vi "TLB Native Dynamic Events ver 0.02.vi"() -> ()   [LabVIEW 2018]
uses:
  Labview Training Phase 2/Enum Controls/States for Action Engine.ctl
panel:
  out "QUEUE OUTPUT":string
  in  "Stop Queue":bool
  in  "Start Queue":bool
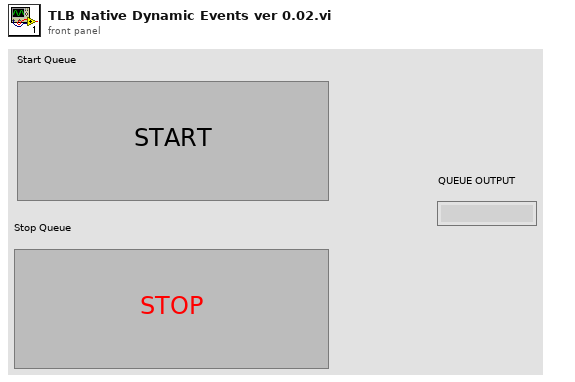
[diagram p1: front panel]
types:
  T1 = typedef "States for Action Engine.ctl" = enum16{"Initialize", "Write", "Read"}
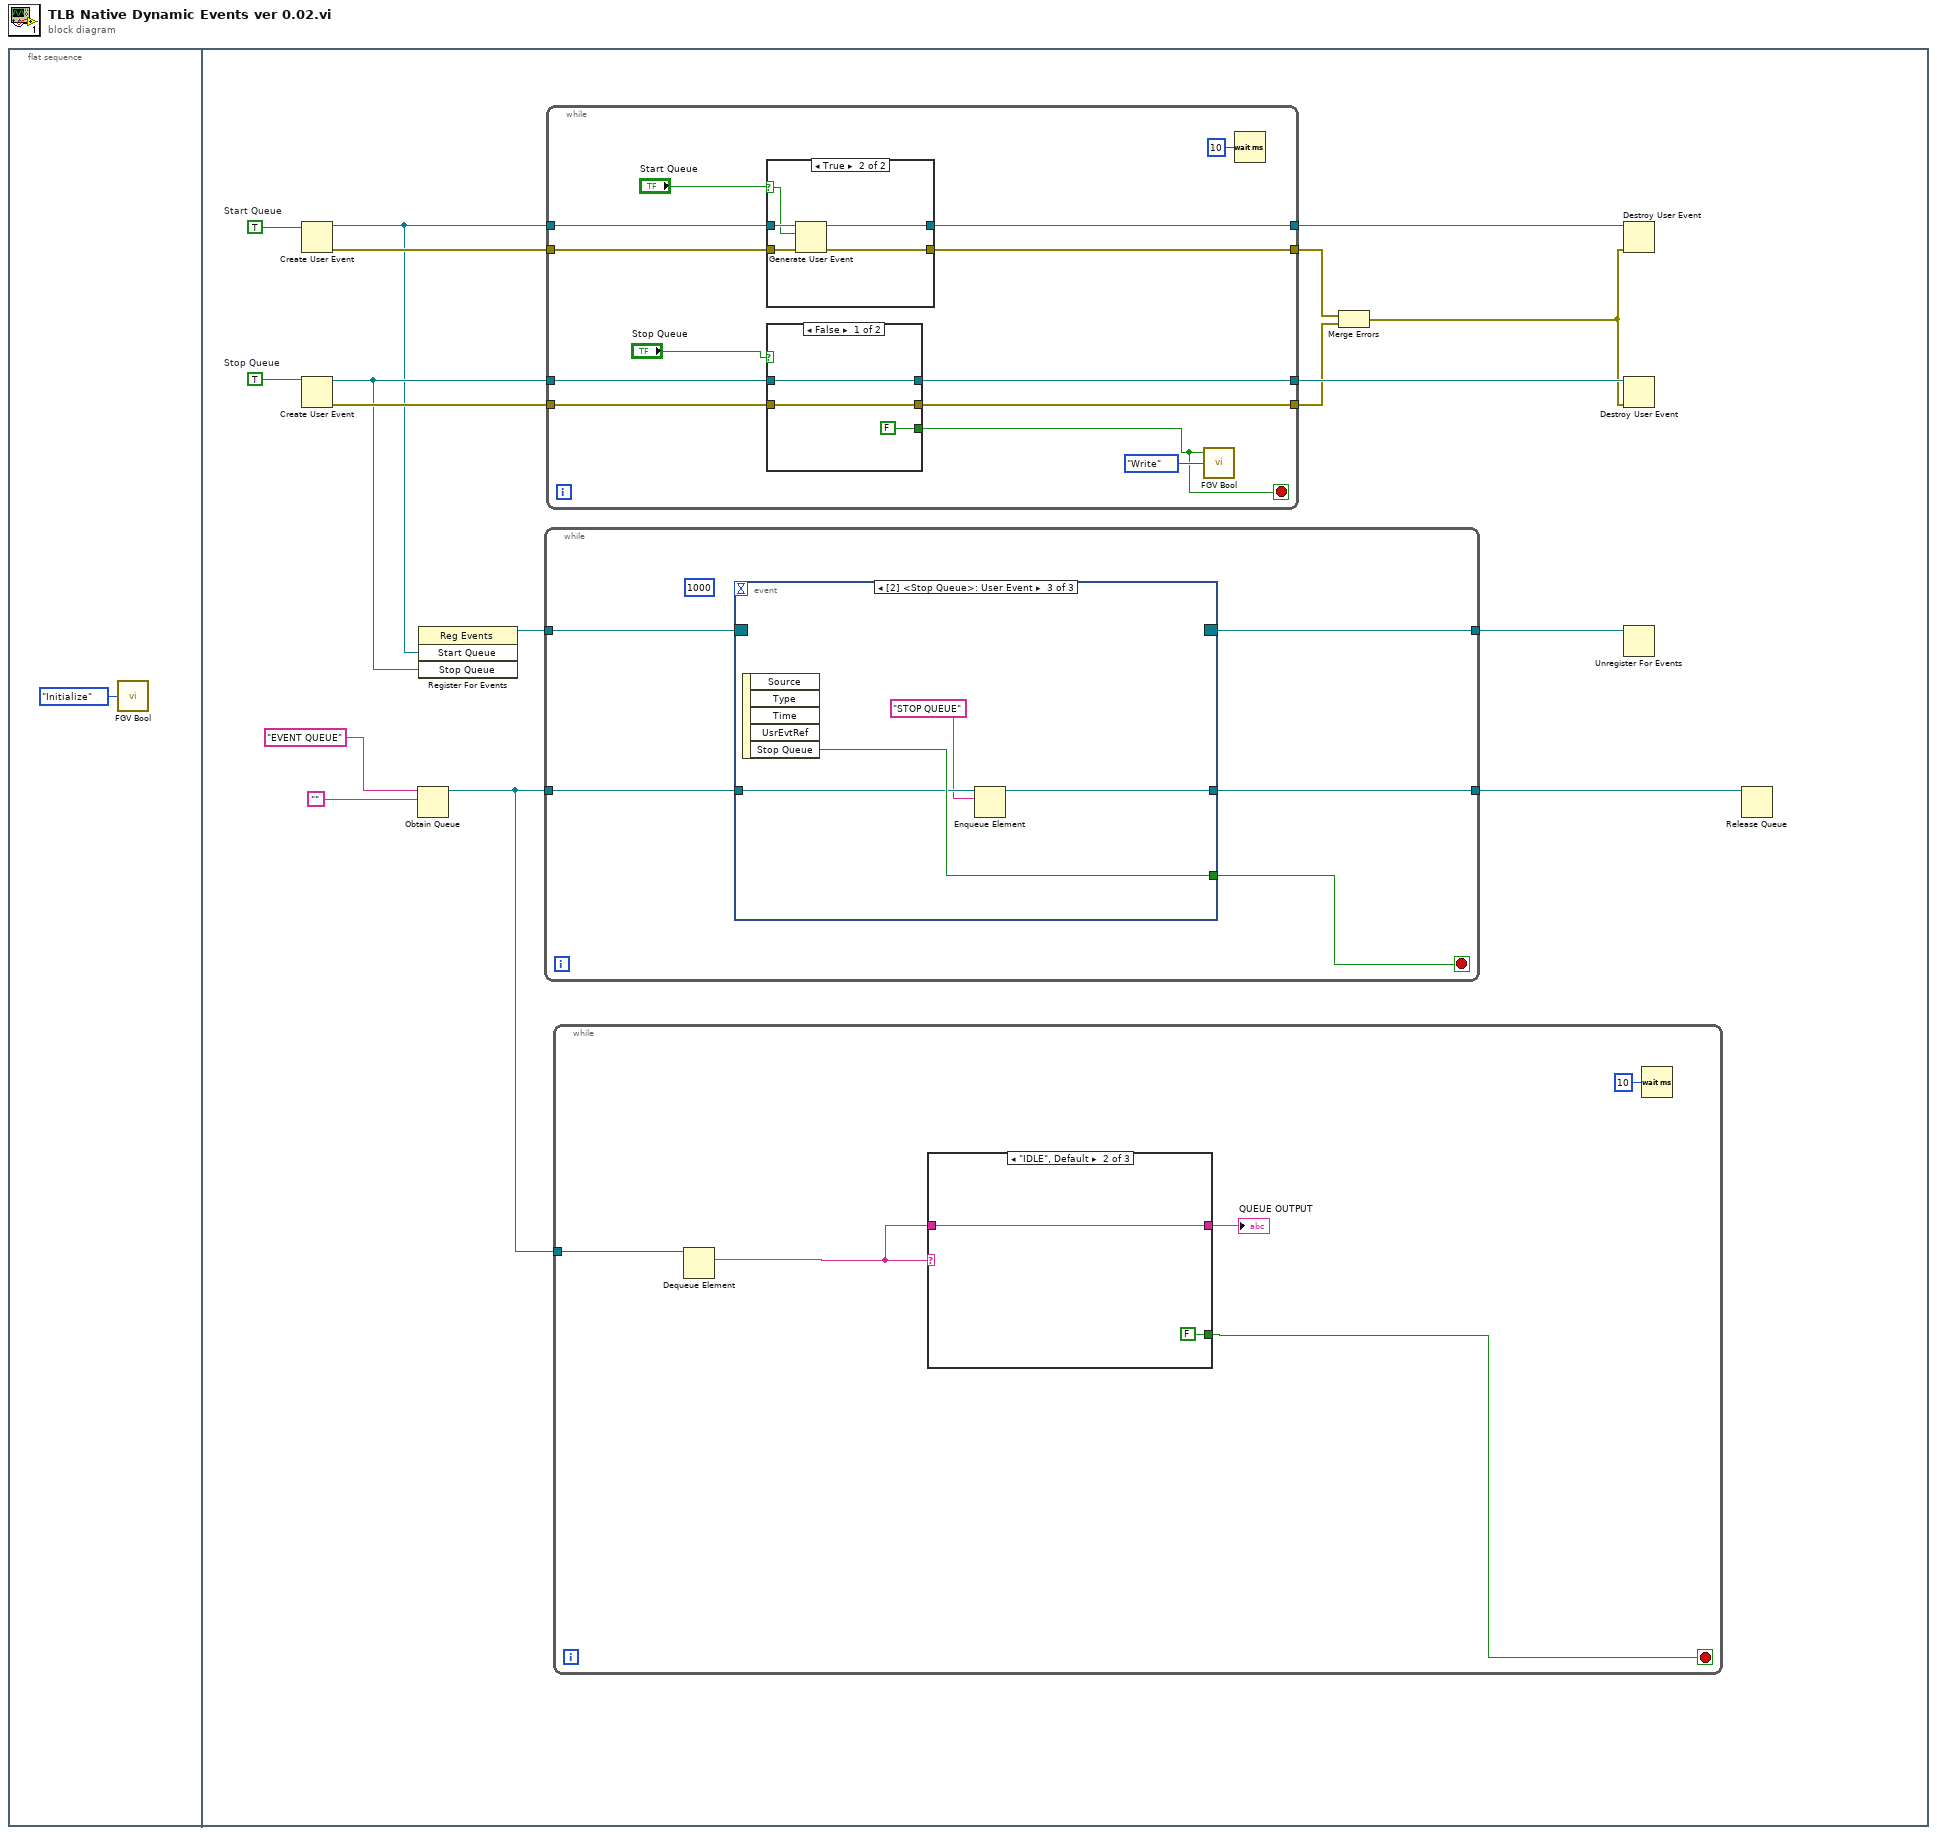
[diagram p0: block diagram]
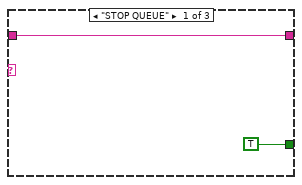
[diagram p2: hidden frame]
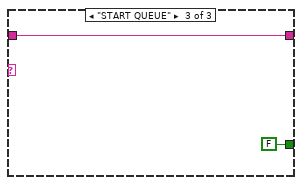
[diagram p3: hidden frame]
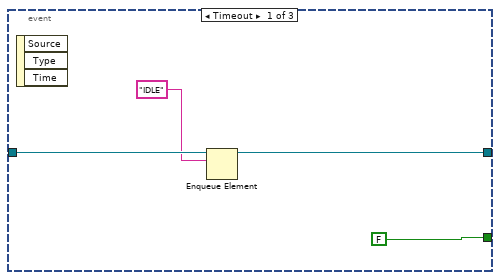
[diagram p4: hidden frame]
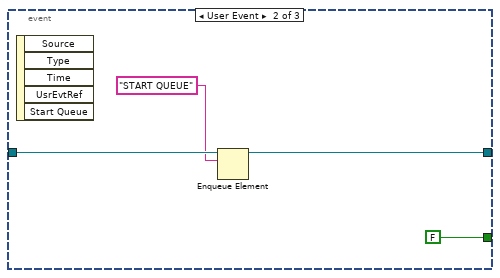
[diagram p5: hidden frame]
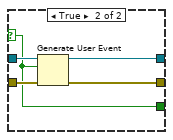
[diagram p6: hidden frame]
diagram:
  n1 = flat-sequence {
    frame #0 {
      n2 = call "FGV Bool.vi"("Init/Read/Write State"=States_for_Action_Engine."Initialize") -> ()  [unwired: 2 in, 2 out]
    }
    frame #1 {
      w18 = TRUE  # Stop Queue
      w17 = TRUE  # Start Queue
      n3 = Create User Event(user event datatype=w17) -> (user event=w8:refnum<user-event>, error out=w14:errorcluster)  [unwired: 1 in]
      n4 = Create User Event(user event datatype=w18) -> (user event=w9:refnum<user-event>, error out=w13:errorcluster)  [unwired: 1 in]
      n5 = Obtain Queue(name (unnamed)="EVENT QUEUE", element data type="") -> (queue out=w2:refnum<queue>)  [unwired: 3 in, 2 out]
      n6 = register-events(w8, w9) -> (reference out=w7:refnum<event-registration>)  [unwired: 2 in, 1 out]
      n7 = while {
        tunnel: w7 -> [w34]
        tunnel: [w33] -> w6
        tunnel: w2 -> [w31]
        tunnel: [w30] -> w5
        stop <- w32 stop-if-true
        (unwired) 1000
        n8 = event shown="[2] <Stop Queue>: User Event" {
          selector: w34 -> [_ _ _]
          dyn-events: [_ _ _] -> w33
          timeout: _ -> [_ _ _]
          tunnel: [FALSE FALSE w46] -> w32
          tunnel: w31 -> [w37 w41 w44]
          tunnel: [w36 w40 w45] -> w30
          event Timeout {
            n9 = event-data() -> ()  [unwired: 1 in, 3 out]
            n10 = Enqueue Element(queue=w37, element="IDLE") -> (queue out=w36:refnum<queue>)  [unwired: 2 in, 2 out]
          }
          event User Event {
            n11 = event-data() -> ()  [unwired: 1 in, 5 out]
            n12 = Enqueue Element(queue=w41, element="START QUEUE" ("name (unnamed)")) -> (queue out=w40:refnum<queue>)  [unwired: 2 in, 2 out]
          }
          event User Event {
            n13 = event-data() -> ("Stop Queue"=w46:bool)  [unwired: 1 in, 4 out]
            n14 = Enqueue Element(queue=w44, element="STOP QUEUE") -> (queue out=w45:refnum<queue>)  [unwired: 2 in, 2 out]
          }
        }
      }
      n15 = while {
        tunnel: w8 -> [w58]
        tunnel: w9 -> [w57]
        tunnel: [w56] -> w16
        tunnel: [w55] -> w15
        tunnel: w14 -> [w54]
        tunnel: [w53] -> w12
        tunnel: w13 -> [w52]
        tunnel: [w51] -> w11
        stop <- w47 stop-if-true
        n16 = case shown="True" "Start Queue" {
          selector: "Start Queue" -> [_ w70]
          tunnel: w58 -> [w69 w74]
          tunnel: [w69 w73] -> w55
          tunnel: w54 -> [w68 w72]
          tunnel: [w68 w71] -> w53
          frame False {
          }
          frame True {
            n17 = Generate User Event(user event=w74, event data cluster=w70, error in=w72) -> (user event out=w73:refnum<user-event>, error out=w71:errorcluster)  [unwired: 1 in]
          }
        }
        n18 = case shown="False" "Stop Queue" {
          selector: "Stop Queue" -> [_ w63]
          tunnel: w57 -> [w62 w67]
          tunnel: [w62 w66] -> w56
          tunnel: w52 -> [w61 w65]
          tunnel: [w61 w64] -> w51
          tunnel: [FALSE w63] -> w47
          frame False {
          }
          frame True {
            n19 = Generate User Event(user event=w67, event data cluster=w63, error in=w65) -> (user event out=w66:refnum<user-event>, error out=w64:errorcluster)  [unwired: 1 in]
          }
        }
        n20 = call "FGV Bool.vi"("Init/Read/Write State"=States_for_Action_Engine."Write", "Input Node"=w47) -> ()  [unwired: 1 in, 2 out]
        n21 = Wait (ms)(milliseconds to wait=u32 10) -> ()  [unwired: 1 out]
      }
      n22 = while {
        tunnel: w2 -> [w23]
        stop <- w19 stop-if-true
        n23 = Dequeue Element(queue=w23) -> (element=w22:string)  [unwired: 2 in, 3 out]
        n24 = case shown="\"IDLE\", Default" w22 {
          tunnel: w22 -> [w25 w27 w29]
          tunnel: [w25 w27 w29] -> w21
          tunnel: [TRUE FALSE FALSE] -> w19
          frame "STOP QUEUE" {
          }
          frame "IDLE", Default {
          }
          frame "START QUEUE" {
          }
        }
        "QUEUE OUTPUT" <- w21
        n25 = Wait (ms)(milliseconds to wait=u32 10) -> ()  [unwired: 1 out]
      }
      n26 = Merge Errors(w12, w11) -> (w10:errorcluster)
      n27 = Destroy User Event(user event=w15, error in=w10) -> ()  [unwired: 1 out]
      n28 = Destroy User Event(user event=w16, error in=w10) -> ()  [unwired: 1 out]
      n29 = Unregister For Events(event registration refnum=w6) -> ()  [unwired: 1 in, 1 out]
      n30 = Release Queue(queue=w5) -> ()  [unwired: 2 in, 3 out]
    }
  }
